vi "Contr_Receive.vi"(4 "error in":errorcluster, 5 "Command to SIFS":string, 6 "wait after tx":u32, 7 "VISA resource name":refnum<visa-resource-name>) -> (0 "error out":errorcluster, 1 "cmd sent":bool, 2 "Response from SIFS":string, 3 "VISA resource name out":refnum<visa-resource-name>)   [LabVIEW 2012]
uses:
  GLOBAL.vi
panel:
  out "Serial Settings:Number of Bytes at Serial Port":u32
  out "error out 5":errorcluster
  out "error out 4":errorcluster
  out "LIXO":string
  out "error out 3":errorcluster
  out "error out 2":errorcluster
  out "error IO":errorcluster
  out "Numeric":i32
  out "read buffer":string
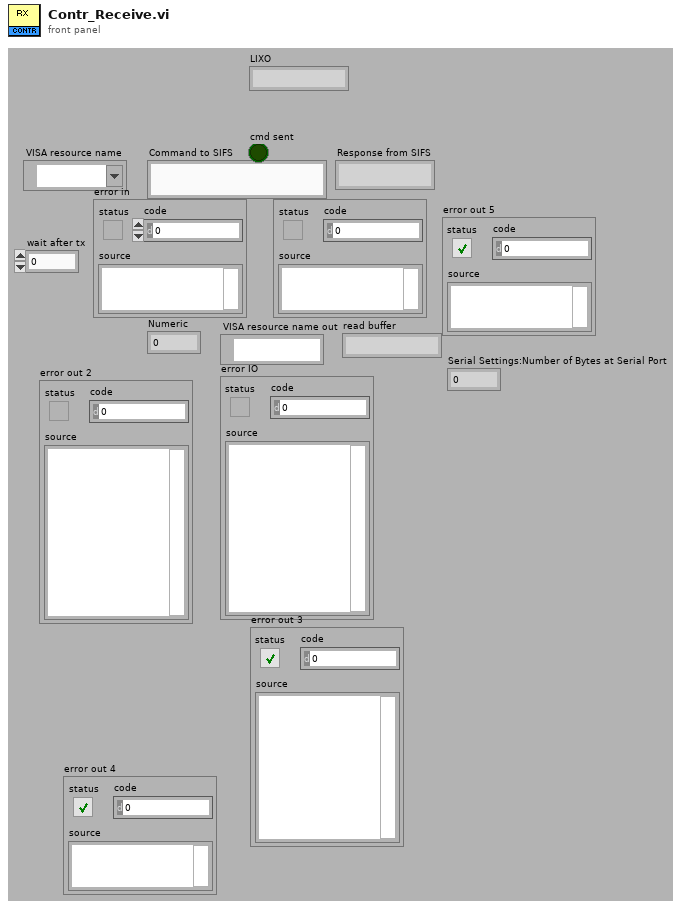
[diagram p1: front panel]
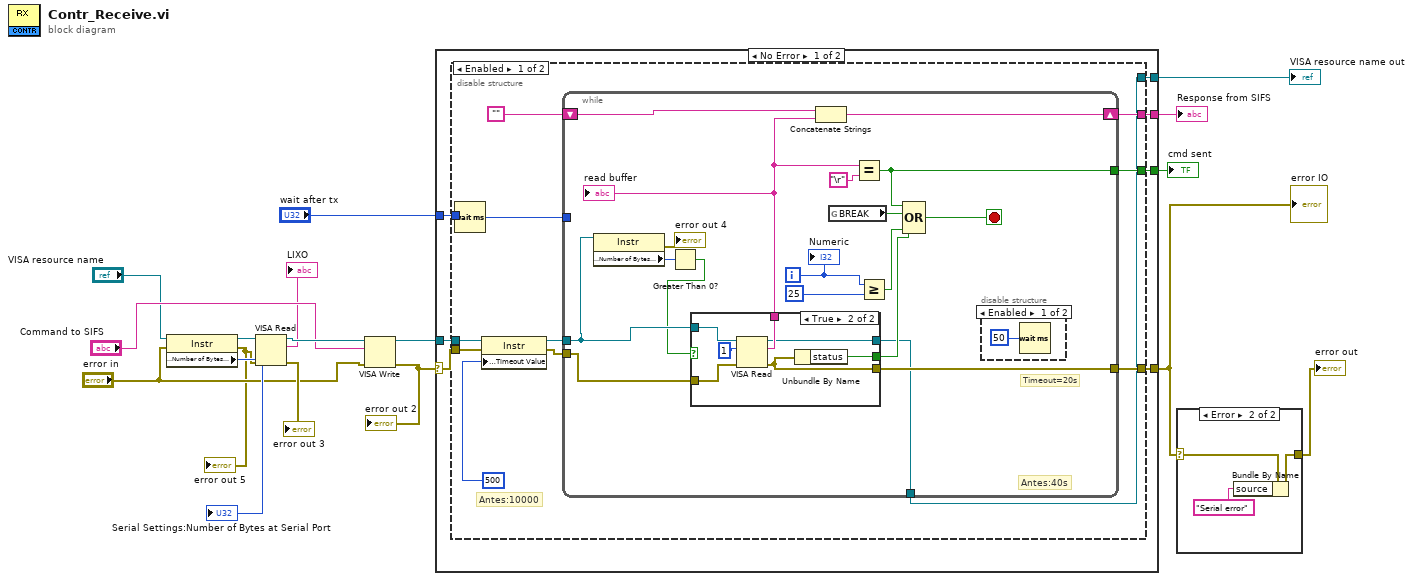
[diagram p0: block diagram]
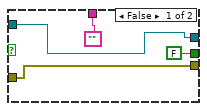
[diagram p3: hidden frame]
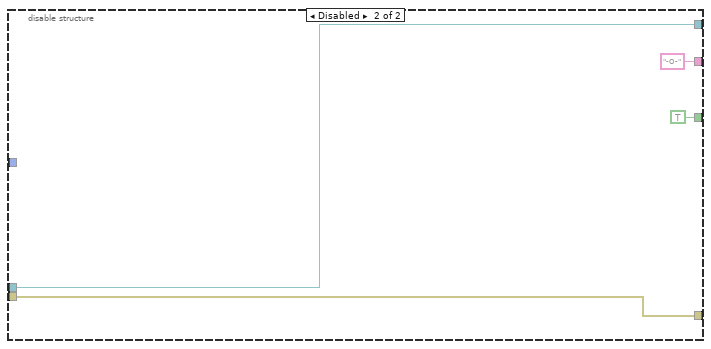
[diagram p5: hidden frame]
diagram:
  n1 = property class="Instr"(reference="VISA resource name", error in="error in") -> (reference out=w8:refnum<visa-resource-name>, error out=w3:errorcluster, "Serial Settings:Number of Bytes at Serial Port"=w7:u32)
  "error out 5" <- w3
  "Serial Settings:Number of Bytes at Serial Port" <- w7
  n2 = VISA Read(VISA resource name=w8, byte count=w7, error in (no error)=w3) -> (VISA resource name out=w6:refnum<visa-resource-name>, read buffer=→"LIXO":string, error out=→"error out 3":errorcluster)  [unwired: 1 out]
  n3 = VISA Write(VISA resource name=w6, write buffer="Command to SIFS", error in (no error)="error in") -> (VISA resource name out=w16:refnum<visa-resource-name>, error out=w15:errorcluster)  [unwired: 1 out]
  "error out 2" <- w15
  n4 = case shown="No Error" w15 {
    selector: w15 -> [w19 w72]
    tunnel: [w22 w72] -> w13
    tunnel: [w24 _] -> w17
    tunnel: w16 -> [w20 w71]
    tunnel: "wait after tx" -> [w23 _]
    tunnel: [w21 _] -> w11
    tunnel: [w18 w71] -> w10
    frame No Error {
      n5 = disable-structure shown="Enabled" {
        disable-tunnel: [w36 "-O-"] -> w24
        disable-tunnel: w23 -> [w33 _]
        disable-tunnel: [w32 w70] -> w22
        disable-tunnel: [w31 TRUE] -> w21
        disable-tunnel: w20 -> [w29 w69]
        disable-tunnel: w19 -> [w26 w70]
        disable-tunnel: [w25 w69] -> w18
        frame Enabled {
          # "Antes:10000"
          n6 = Wait (ms)(milliseconds to wait=w33) -> (millisecond timer value=w34:u32)
          n7 = property class="Instr"(reference=w29, error in=w26, "General Settings:Timeout Value"=u32 500) -> (reference out=w28:refnum<visa-resource-name>, error out=w27:errorcluster)
          n8 = while {
            shift-right: [w53] -> w36
            shift-left: "" -> [w54]
            tunnel: [w45] -> w32
            tunnel: w34 -> [_]
            tunnel: [w44] -> w31
            tunnel: w28 -> [w40]
            tunnel: w27 -> [w43]
            tunnel: [w42] -> w25
            i -> [w49]
            stop <- w50 stop-if-true
            # "Antes:40s"
            # "Timeout=20s"
            n9 = property class="Instr"(reference=w40) -> (error out=→"error out 4":errorcluster, "Serial Settings:Number of Bytes at Serial Port"=w39:u32)  [unwired: 1 in, 1 out]
            n10 = Greater Than 0?(x=w39) -> (x > 0?=w38:bool)
            n11 = case shown="True" w38 {
              tunnel: ["" w64] -> w52
              tunnel: [FALSE ("status") w63] -> w46
              tunnel: [w56 w62] -> w45
              tunnel: w40 -> [w57 w61]
              tunnel: w43 -> [w56 w60]
              tunnel: [w57 w59] -> w42
              frame False {
              }
              frame True {
                n12 = VISA Read(VISA resource name=w61, byte count=u32 1, error in (no error)=w60) -> (VISA resource name out=w59:refnum<visa-resource-name>, read buffer=w64:string, error out=w62:errorcluster)  [unwired: 1 out]
                n13 = Unbundle By Name(w62) -> ("status"=w63:bool)
              }
            }
            "read buffer" <- w52
            n14 = Concatenate Strings(w54, w52) -> (w53:string)
            n15 = global read "GLOBAL.vi" "BREAK"() -> (w51:bool)
            n16 = Equal?(x=w52, y="\r") -> (x = y?=w44:bool)
            n17 = Greater Or Equal?(x=w49, y=25) -> (x >= y?=w47:bool)
            n18 = Compound Arithmetic op=OR(w44, w51, w47, w46) -> (w50:bool)
            n19 = disable-structure shown="Enabled" {
              frame Enabled {
                n20 = Wait (ms)(milliseconds to wait=u32 50 ("millisecond multiple")) -> ()  [unwired: 1 out]
              }
              frame Disabled {
              }
            }
            "Numeric" <- w49
          }
        }
        frame Disabled {
        }
      }
    }
    frame Error {
    }
  }
  "Response from SIFS" <- w17
  "VISA resource name out" <- w10
  "cmd sent" <- w11
  "error IO" <- w13
  n21 = case shown="Error" w13 {
    selector: w13 -> [w73 w75]
    tunnel: [w73 w74] -> w12
    frame No Error {
    }
    frame Error {
      n22 = Bundle By Name(cluster=w75, "source"="Serial error") -> (w74:errorcluster)
    }
  }
  "error out" <- w12
